vi "Read ILC Settings.vi"(8 "error in (no error)":errorcluster, 11 "Boot Loader in":refnum<class "Boot Loader.lvclass">) -> (0 "error out":errorcluster, 1 "Serial Settings":T1={"Baud Rate"=9600, "Data Bits"=8, "Parity"=enum."None", "Flow Control"=0, "Stop Bits"=10, "Timeout (ms)"=10000, "Byte Count"=200, "Enable Termination Character"=FALSE, "Termination Char"=200} {"Termination Char" format="%x"; "Stop Bits" items=["1.0"=10, "1.5"=15, "2.0"=20]; "Flow Control" items=["None", "XON/XOFF", "RTS/CTS", "XON/XOFF & RTS/CTS", "DTR/DSR", "XON/XOFF & DTR/DSR"]; "Data Bits" min=5 max=8 step=1}, 2 "ILC Port":refnum<visa-resource-name>, 3 "Boot Loader out":refnum<class "Boot Loader.lvclass">)   [LabVIEW 2016, in "Boot Loader.lvclass"]
uses:
  Boot Loader.lvclass
  Typedefs/SerialSettings.ctl
  Typedefs/HPMT_Typedefs.lvlib
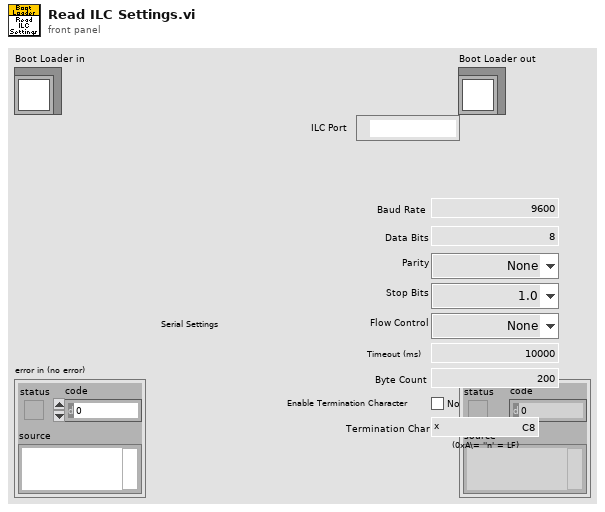
[diagram p1: front panel]
types:
  T1 = typedef "HPMT_Typedefs.lvlib/SerialSettings.ctl" = cluster{"Baud Rate":u32, "Data Bits":u16, "Parity":enum16{"None", "Odd", "Even", "Mark", "Space"}, "Flow Control":u16, "Stop Bits":u16, "Timeout (ms)":u32, "Byte Count":u32, "Enable Termination Character":bool, "Termination Char":u8}
  T2 = typedef "M1M3SupportEUI_TypeDefs.lvlib/ConnectionSettings.ctl" = cluster{"ILC Port":refnum<visa-resource-name>}
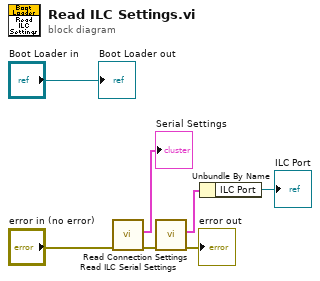
[diagram p0: block diagram]
diagram:
  n1 = call "Read ILC Serial Settings.vi"("error in (no error)"="error in (no error)") -> ("error out"=w3:errorcluster, "Serial Settings"=→"Serial Settings":T1)  [unwired: 8 in, 1 out]
  n2 = call "Read Connection Settings.vi"("error in (no error)"=w3) -> ("error out"=→"error out":errorcluster, "Connection Settings"=w7:T2)  [unwired: 8 in, 1 out]
  n3 = Unbundle By Name(w7) -> ("ILC Port"=→"ILC Port":refnum<visa-resource-name>)
  "Boot Loader out" <- "Boot Loader in"
